vi "Grid_Scan_Stiching.vi"() -> ()   [LabVIEW 2014]
uses:
  shared/CorrelImages (SubVI)Single.vi
  <userlib>/Nanonis Prog Interface V5/Nanonis Prog Interface.lvlib
panel:
  out "Size (m) 3":cluster{"Width":sgl, "Height":sgl} {"Height" format="%.2p"; "Width" format="%.2p"}
  in  "Size (m) 2":cluster{"Width":sgl, "Height":sgl} {"Height" format="%.2p"; "Width" format="%.2p"}
  in  "Large Grid Size(m)":dbl format="%#_6p"
  in  "Tip Speed (m/s)":sgl=1e-08 format="%.2p"
  in  "Set Bias Timing (ms)":i32
  out "Grid Size 2":cluster{"Width":sgl, "Height":sgl}
  in  "Overlap (m)":dbl format="%#_6p"
  in  "Overlap (m)":cluster{"Width":sgl, "Height":sgl}
  in  "Pixels":i32 caption="Pixels/line"
  in  "Grid Coordinates":cluster{"Xc":sgl, "Yc":sgl} {"Yc" format="%.2p"; "Xc" format="%.2p"}
  out "floor(x/y)":i32
  out "yi":i32
  in  "img delay (s)":u32=1
  in  "TipLift (m)":sgl format="%#_6p"
  out "timing":i32
  out "Grid Size":cluster{"Width":sgl, "Height":sgl}
  out "Angle (deg)":sgl format="%.2f"
  out "Size (m)":cluster{"Width":sgl, "Height":sgl} {"Height" format="%.2p"; "Width" format="%.2p"}
  out "Center coordinates (m)":cluster{"Xc":sgl, "Yc":sgl} {"Yc" format="%.2p"; "Xc" format="%.2p"}
  in  "# of Grids":i32=1 min=1 max=10
  in  "ref bias":dbl=-0.0012 format="%#_6p"
  out "DC active":bool
  out "Y drift":i32
  out "X drift":i32
  in  "Current":dbl=5e-11 format="%#_6p"
  in  "Bias":dbl=0.02 format="%#_6p"
  in  "Settling time (s)":dbl=0.7 format="%#_6p"
  in  "Channel index (0-23)":u8(ring) items=["Current"=0, "Z (m)"=14]
  in  "Img Speed":sgl=4.5e-08 format="%#_6p"
  in  "Img Bias (V) DC":sgl=1.0 format="%_2p"
  in  "Img Current":sgl=1e-10 format="%#_6p"
  in  "Drift correction Pixels":i32=128
  in  "Forward Speed":sgl=1.2e-09 format="%#_6p"
  in  "Backward Speed":sgl=8e-08 format="%#_6p"
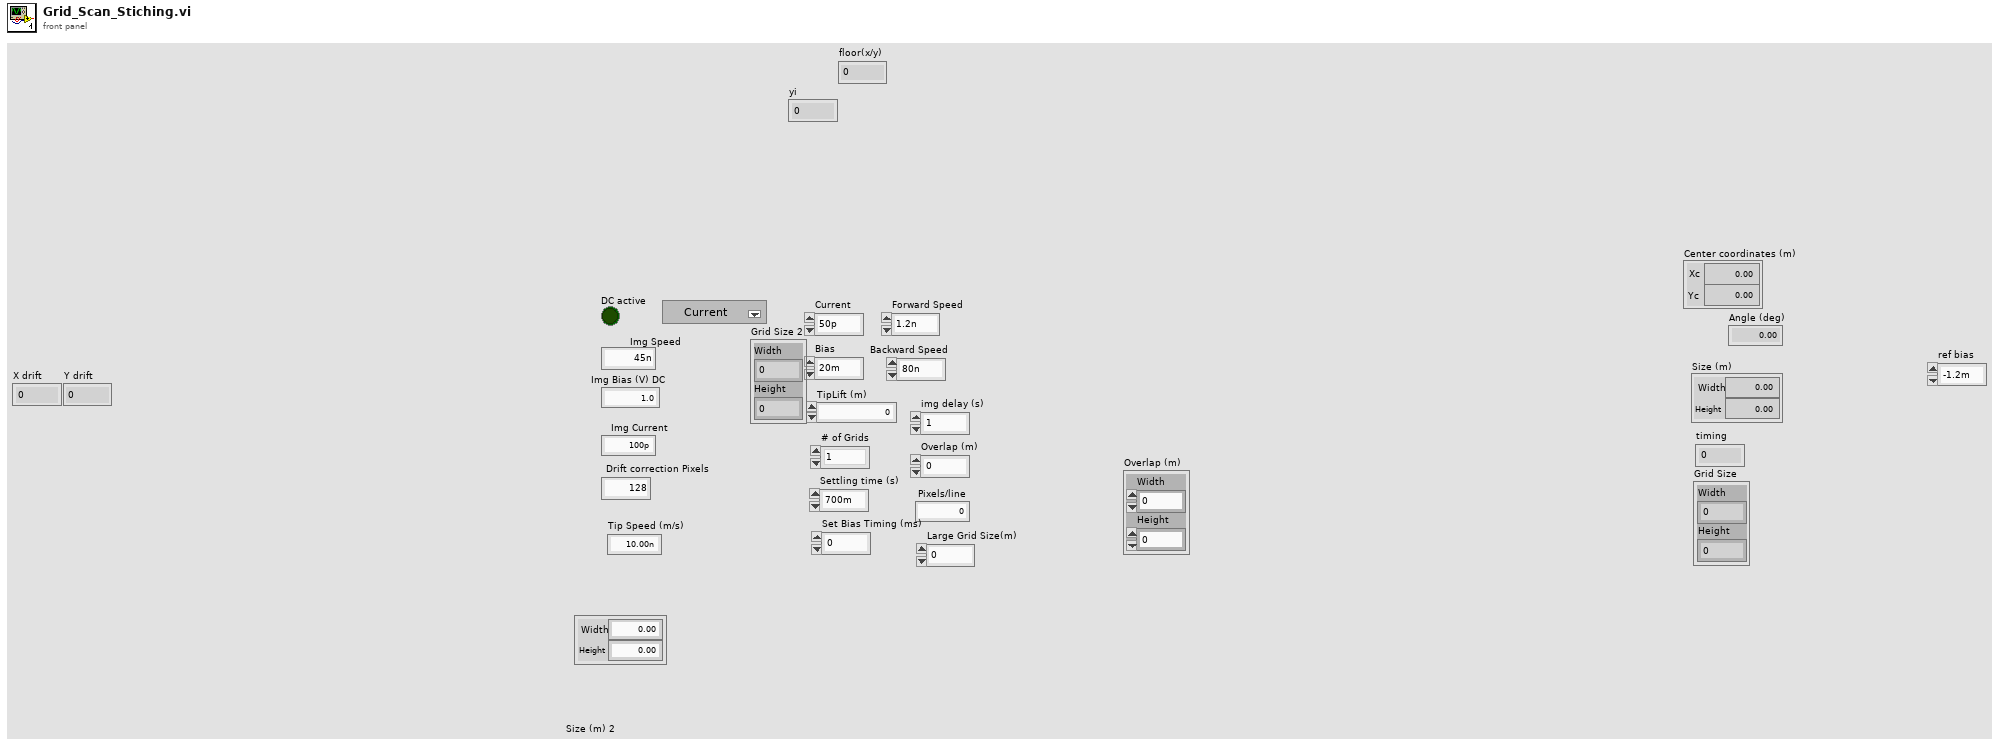
[diagram p1: front panel]
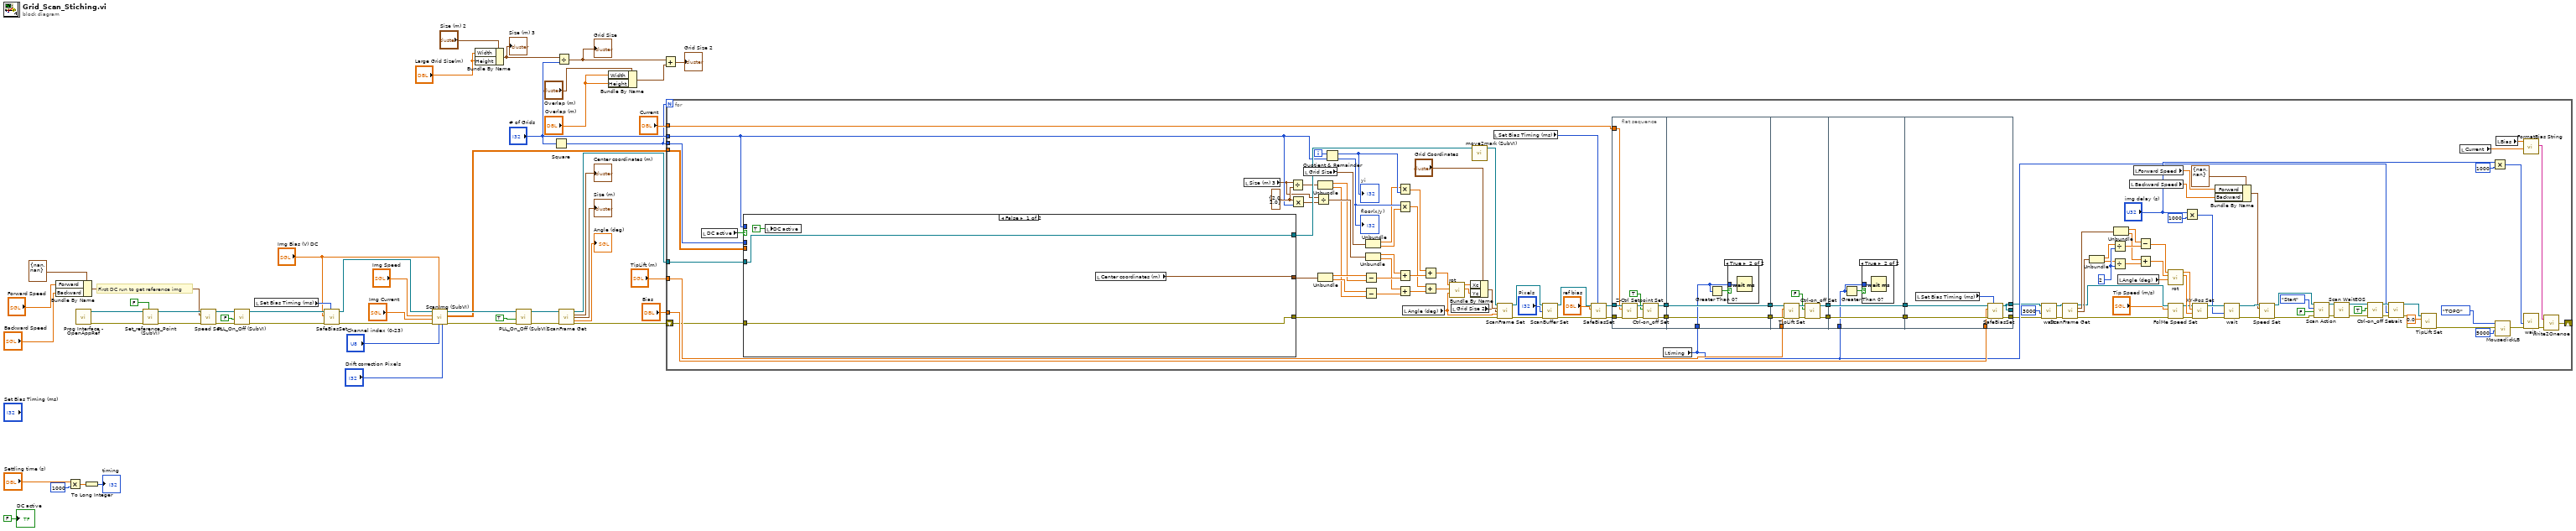
[diagram p0: block diagram]
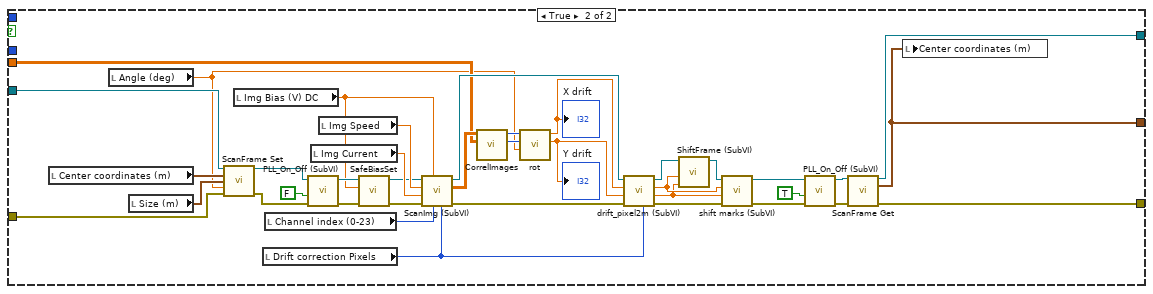
[diagram p2: hidden frame]
diagram:
  # "First DC run to get reference img"
  n1 = Bundle By Name(cluster=cluster{"Forward":sgl, "Backward":sgl} {"Forward"=nan, "Backward"=nan} ("Speed (m/s)"), "Forward"="Forward Speed", "Backward"="Backward Speed") -> (w44:cluster{"Forward":sgl, "Backward":sgl})
  n2 = Multiply(x="Settling time (s)", y=u32 1000) -> (x*y=w28:dbl)
  n3 = call <userlib>:"Prog Interface - OpenAppRef.vi"() -> ("Error out"=w50:errorcluster, "Application reference"=w51:refnum<vi>)  [unwired: 6 in]
  n4 = To Long Integer(number=w28) -> (32bit integer=→"timing":i32)
  n5 = call "Set_reference_Point (SubVI).vi"("Part of multigrid"=FALSE, "error in (no error)"=w50, "Application in"=w51) -> ("error out"=w46:errorcluster, "Application out"=w45:refnum<vi>)  [unwired: 7 in]
  n6 = call <userlib>:"Speed Set.vi"("Application ref in"=w45, "Speed (m/s)"=w44, "error in (no error)"=w46) -> ("Application ref out"=w41:refnum<vi>, "error out"=w42:errorcluster)  [unwired: 11 in]
  n7 = call "PLL_On_Off (SubVI).vi"("error in (no error)"=w42, "Output ON/OFF (F=OFF)"=FALSE, "Application in"=w41) -> ("error out"=w8:errorcluster, "Application out"=w7:refnum<vi>)  [unwired: 7 in]
  n8 = local read "Set Bias Timing (ms)"() -> (w5:i32)
  n9 = call "SafeBiasSet.vi"("Application ref in"=w7, "Bias (V)"="Img Bias (V) DC", "error in (no error)"=w8, "milliseconds to wait"=w5) -> ("Application ref out"=w6:refnum<vi>, "Error out"=w9:errorcluster)  [unwired: 5 in]
  n10 = call "ScanImg (SubVI).vi"("pixel"="Drift correction Pixels", "Channel index (0-23)"="Channel index (0-23)", "Bias (V)"="Img Bias (V) DC", "error in (no error)"=w9, "Current"="Img Current", "Img Speed"="Img Speed", "Application in"=w6) -> ("error out"=w37:errorcluster, "Img"=w10:dbl[][], "Application out"=w38:refnum<vi>)  [unwired: 2 in]
  n11 = Bundle By Name(cluster="Size (m) 2", "Width"="Large Grid Size(m)", "Height"="Large Grid Size(m)") -> (w1:cluster{"Width":sgl, "Height":sgl})
  "Size (m) 3" <- w1
  n12 = call "PLL_On_Off (SubVI).vi"("error in (no error)"=w37, "Output ON/OFF (F=OFF)"=TRUE, "Application in"=w38) -> ("error out"=w32:errorcluster, "Application out"=w33:refnum<vi>)  [unwired: 7 in]
  n13 = Square(x="# of Grids") -> (x^2=w20:i32)
  n14 = Divide(x=w1, y="# of Grids") -> (x/y=w11:cluster{"Width":sgl, "Height":sgl})
  "Grid Size" <- w11
  n15 = call <userlib>:"ScanFrame Get.vi"("Application ref in"=w33, "error in (no error)"=w32) -> ("Application ref out"=w22:refnum<vi>, "Center coordinates (m)"=→"Center coordinates (m)":cluster{"Xc":sgl, "Yc":sgl}, "Size (m)"=→"Size (m)":cluster{"Width":sgl, "Height":sgl}, "Angle (deg)"=→"Angle (deg)":sgl, "error out"=w16:errorcluster)  [unwired: 9 in]
  n16 = Bundle By Name(cluster="Overlap (m)", "Width"="Overlap (m)", "Height"="Overlap (m)") -> (w14:cluster{"Width":sgl, "Height":sgl})
  n17 = Add(x=w11, y=w14) -> (x+y=→"Grid Size 2":cluster{"Width":sgl, "Height":sgl})
  n18 = for {
    N: w20 -> [_]
    tunnel: "TipLift (m)" -> [w162]
    tunnel: "Bias" -> [w161]
    shift-right: [w70] -> _
    shift-left: w16 -> [w117]
    tunnel: "Current" -> [w119]
    tunnel: w22 -> [w115]
    tunnel: "# of Grids" -> [w110]
    tunnel: w20 -> [w114]
    tunnel: w10 -> [w52]
    i -> [w112]
    w111 = cluster{"Width":sgl, "Height":sgl} {"Width"=2.0, "Height"=2.0} ("y")
    w149 = 2
    n19 = local read "DC active"() -> (w74:bool)
    n20 = case shown="False" w74 {
      tunnel: [w176 w186] -> w118
      tunnel: w117 -> [w176 w192]
      tunnel: [w175 w193] -> w116
      tunnel: w115 -> [w175 w191]
      tunnel: w110 -> [_ _]
      tunnel: w114 -> [_ _]
      tunnel: [w174 w178] -> w97
      tunnel: w52 -> [_ w185]
      frame False {
        n21 = local write "DC active"(TRUE ("DC active")) -> ()
        n22 = local read "Center coordinates (m)"() -> (w174:cluster{"Xc":sgl, "Yc":sgl})
      }
      frame True {
        n23 = local read "Center coordinates (m)"() -> (w188:cluster{"Xc":sgl, "Yc":sgl})
        n24 = local read "Angle (deg)"() -> (w179:sgl)
        n25 = local read "Size (m)"() -> (w187:cluster{"Width":sgl, "Height":sgl})
        n26 = call <userlib>:"ScanFrame Set.vi"("Application ref in"=w191, "Center coordinates (m)"=w188, "Size (m)"=w187, "Angle (deg)"=w179, "error in (no error)"=w192) -> ("Application ref out"=w190:refnum<vi>, "error out"=w189:errorcluster)  [unwired: 9 in]
        n27 = local read "Img Bias (V) DC"() -> (w180:sgl)
        n28 = local read "Drift correction Pixels"() -> (w210:i32)
        n29 = local read "Channel index (0-23)"() -> (w206:u8)
        n30 = call "PLL_On_Off (SubVI).vi"("error in (no error)"=w189, "Output ON/OFF (F=OFF)"=FALSE, "Application in"=w190) -> ("error out"=w182:errorcluster, "Application out"=w184:refnum<vi>)  [unwired: 7 in]
        n31 = local read "Img Current"() -> (w205:sgl)
        n32 = local read "Img Speed"() -> (w204:sgl)
        n33 = call "SafeBiasSet.vi"("Application ref in"=w184, "Bias (V)"=w180, "error in (no error)"=w182) -> ("Application ref out"=w183:refnum<vi>, "Error out"=w181:errorcluster)  [unwired: 6 in]
        n34 = call "ScanImg (SubVI).vi"("pixel"=w210, "Channel index (0-23)"=w206, "Bias (V)"=w180, "error in (no error)"=w181, "Current"=w205, "Img Speed"=w204, "Application in"=w183) -> ("error out"=w215:errorcluster, "Img"=w203:dbl[][], "Application out"=w208:refnum<vi>)  [unwired: 2 in]
        n35 = call-poly "CorrelImages.vi"("Ref Array"=w185, "New Image"=w203) -> ("Y drift"=w213:i32, "X drift"=w211:i32)  [unwired: 6 in, 2 out]
        n36 = call "rot.vi"("angle"=w179, "y"=w213, "x"=w211) -> ("y'"=w214:sgl, "x'"=w212:sgl)  [unwired: 7 in]
        "X drift" <- w212
        "Y drift" <- w214
        n37 = call "drift_pixel2m (SubVI).vi"("Application in"=w208, "X drift"=w212, "Y drift"=w214, "error in"=w215, "Drift correction Pixels"=w210) -> ("Application out"=w207:refnum<vi>, "x drift"=w201:sgl, "y drift"=w200:sgl, "error out"=w199:errorcluster)  [unwired: 1 in]
        n38 = call "ShiftFrame (SubVI).vi"("Y shift"=w200, "X shift"=w201, "Application in"=w207) -> ("Application out"=w202:refnum<vi>)  [unwired: 8 in]
        n39 = call "shift marks (SubVI).vi"("error in (no error)"=w199, "y"=w200, "x"=w201, "Application in"=w202) -> ("error out"=w197:errorcluster, "Application out"=w198:refnum<vi>)  [unwired: 6 in]
        n40 = call "PLL_On_Off (SubVI).vi"("error in (no error)"=w197, "Output ON/OFF (F=OFF)"=TRUE, "Application in"=w198) -> ("error out"=w194:errorcluster, "Application out"=w195:refnum<vi>)  [unwired: 7 in]
        n41 = call <userlib>:"ScanFrame Get.vi"("Application ref in"=w195, "error in (no error)"=w194) -> ("Application ref out"=w193:refnum<vi>, "Center coordinates (m)"=w178:cluster{"Xc":sgl, "Yc":sgl}, "error out"=w186:errorcluster)  [unwired: 9 in, 2 out]
        n42 = local write "Center coordinates (m)"(w178) -> ()
      }
    }
    n43 = local read "Size (m) 3"() -> (w108:cluster{"Width":sgl, "Height":sgl})
    n44 = Divide(x=w108, y=w111) -> (x/y=w113:cluster{"Width":sgl, "Height":sgl})
    n45 = Multiply(x=w111, y=w110) -> (x*y=w109:cluster{"Width":sgl, "Height":sgl})
    n46 = local read "Grid Size"() -> (w83:cluster{"Width":sgl, "Height":sgl})
    n47 = Divide(x=w108, y=w109) -> (x/y=w107:cluster{"Width":sgl, "Height":sgl})
    n48 = Unbundle(w113) -> ("Width"=w103:sgl, "Height"=w101:sgl)
    n49 = Unbundle(w97) -> ("Xc"=w104:sgl, "Yc"=w102:sgl)
    n50 = Quotient & Remainder(x=w112, y=w110) -> (x-y*floor(x/y)=w105:i32, floor(x/y)=w106:i32)
    "yi" <- w105
    "floor(x/y)" <- w106
    n51 = Subtract(x=w104, y=w103) -> (x-y=w100:sgl)
    n52 = Subtract(x=w102, y=w101) -> (x-y=w99:sgl)
    n53 = Unbundle(w83) -> ("Width"=w82:sgl, "Height"=w81:sgl)
    n54 = Unbundle(w107) -> ("Width"=w85:sgl, "Height"=w84:sgl)
    n55 = Multiply(x=w82, y=w105) -> (x*y=w78:sgl)
    n56 = Multiply(x=w106, y=w81) -> (x*y=w75:sgl)
    n57 = Add(x=w85, y=w100) -> (x+y=w79:sgl)
    n58 = Add(x=w84, y=w99) -> (x+y=w76:sgl)
    n59 = local read "Angle (deg)"() -> (w94:sgl)
    n60 = Add(x=w78, y=w79) -> (x+y=w80:sgl)
    n61 = Add(x=w75, y=w76) -> (x+y=w77:sgl)
    n62 = call "rot.vi"("angle"=w94, "y"=w77, "x"=w80) -> ("y'"=w95:sgl, "x'"=w96:sgl)  [unwired: 7 in]
    n63 = local read "Grid Size 2"() -> (w127:cluster{"Width":sgl, "Height":sgl})
    n64 = Bundle By Name(cluster="Grid Coordinates", "Xc"=w96, "Yc"=w95) -> (w128:cluster{"Xc":sgl, "Yc":sgl})
    n65 = call "move2mark (SubVI).vi"("Application in"=w116) -> ("Application out"=w129:refnum<vi>)  [unwired: 10 in]
    n66 = local read "Set Bias Timing (ms)"() -> (w58:i32)
    n67 = call <userlib>:"ScanFrame Set.vi"("Application ref in"=w129, "Center coordinates (m)"=w128, "Size (m)"=w127, "Angle (deg)"=w94, "error in (no error)"=w118) -> ("Application ref out"=w63:refnum<vi>, "error out"=w60:errorcluster)  [unwired: 9 in]
    n68 = call <userlib>:"ScanBuffer Set.vi"("Application ref in"=w63, "Pixels"="Pixels", "error in (no error)"=w60) -> ("Application ref out"=w62:refnum<vi>, "error out"=w61:errorcluster)  [unwired: 11 in]
    n69 = call "SafeBiasSet.vi"("Application ref in"=w62, "Bias (V)"="ref bias", "error in (no error)"=w61, "milliseconds to wait"=w58) -> ("Application ref out"=w164:refnum<vi>, "Error out"=w165:errorcluster)  [unwired: 5 in]
    n70 = flat-sequence {
      tunnel: [w222] -> w173
      tunnel: [w219] -> w172
      tunnel: w164 -> [w218]
      tunnel: w165 -> [w217]
      tunnel: w119 -> [w216]
      tunnel: w173 -> [w227]
      tunnel: [w227] -> w171
      tunnel: w132 -> [w225]
      tunnel: [w224] -> w170
      tunnel: w172 -> [w224]
      tunnel: w171 -> [w236]
      tunnel: [w234] -> w169
      tunnel: w170 -> [w233]
      tunnel: [w231] -> w168
      tunnel: w162 -> [w229]
      tunnel: w169 -> [w240]
      tunnel: [w240] -> w167
      tunnel: [w238] -> w166
      tunnel: w168 -> [w238]
      tunnel: w132 -> [w237]
      tunnel: [w243] -> _
      tunnel: w167 -> [w247]
      tunnel: w166 -> [w246]
      tunnel: [w245] -> w131
      tunnel: w161 -> [w244]
      tunnel: [w243] -> w130
      frame #0 {
        n71 = call <userlib>:"Z-Ctrl Setpoint Set.vi"("error in (no error)"=w217, "Z Controller setpoint"=w216, "Application ref in"=w218) -> ("error out"=w220:errorcluster, "Application ref out"=w223:refnum<vi>)  [unwired: 7 in]
        n72 = call <userlib>:"Ctrl-on_off Set.vi"("error in (no error)"=w220, "Z Controller ON/OFF"=TRUE, "Application ref in"=w223) -> ("error out"=w219:errorcluster, "Application ref out"=w222:refnum<vi>)  [unwired: 7 in]
      }
      frame #1 {
        n73 = Greater Than 0?(x=w225) -> (x > 0?=w226:bool)
        n74 = case shown="True" w226 {
          tunnel: w225 -> [_ w228]
          frame False {
          }
          frame True {
            n75 = Wait (ms)(milliseconds to wait=w228) -> ()  [unwired: 1 out]
          }
        }
      }
      frame #2 {
        n76 = call <userlib>:"TipLift Set.vi"("error in (no error)"=w233, "TipLift (m)"=w229, "Application ref in"=w236) -> ("error out"=w232:errorcluster, "Application ref out"=w235:refnum<vi>)  [unwired: 7 in]
        n77 = call <userlib>:"Ctrl-on_off Set.vi"("error in (no error)"=w232, "Z Controller ON/OFF"=FALSE, "Application ref in"=w235) -> ("error out"=w231:errorcluster, "Application ref out"=w234:refnum<vi>)  [unwired: 7 in]
      }
      frame #3 {
        n78 = Greater Than 0?(x=w237) -> (x > 0?=w239:bool)
        n79 = case shown="True" w239 {
          tunnel: w237 -> [_ w241]
          frame False {
          }
          frame True {
            n80 = Wait (ms)(milliseconds to wait=w241) -> ()  [unwired: 1 out]
          }
        }
      }
      frame #4 {
        n81 = local read "Set Bias Timing (ms)"() -> (w242:i32)
        n82 = call "SafeBiasSet.vi"("Application ref in"=w247, "Bias (V)"=w244, "error in (no error)"=w246, "milliseconds to wait"=w242) -> ("Application ref out"=w243:refnum<vi>, "Error out"=w245:errorcluster)  [unwired: 5 in]
      }
    }
    n83 = local read "timing"() -> (w132:i32)
    n84 = call "wait.vi"("error in"=w131, "milliseconds to wait"=u32 3000 ("y"), "application reference in"=w130) -> ("error out"=w141:errorcluster, "application reference out"=w140:refnum<vi>)  [unwired: 7 in]
    n85 = call <userlib>:"ScanFrame Get.vi"("Application ref in"=w140, "error in (no error)"=w141) -> ("Application ref out"=w57:refnum<vi>, "Center coordinates (m)"=w144:cluster{"Xc":sgl, "Yc":sgl}, "Size (m)"=w145:cluster{"Width":sgl, "Height":sgl}, "error out"=w56:errorcluster)  [unwired: 9 in, 1 out]
    n86 = Unbundle(w145) -> ("Width"=w147:sgl, "Height"=w148:sgl)
    n87 = Divide(x=w147, y=w149) -> (x/y=w151:sgl)
    n88 = Divide(x=w148, y=w149) -> (x/y=w150:sgl)
    n89 = Unbundle(w144) -> ("Xc"=w152:sgl, "Yc"=w146:sgl)
    n90 = local read "Angle (deg)"() -> (w124:sgl)
    n91 = local read "Backward Speed"() -> (w87:sgl)
    n92 = local read "Forward Speed"() -> (w86:sgl)
    n93 = Subtract(x=w152, y=w151) -> (x-y=w126:sgl)
    n94 = Add(x=w146, y=w150) -> (x+y=w125:sgl)
    n95 = call "rot.vi"("angle"=w124, "y"=w125, "x"=w126) -> ("y'"=w122:sgl, "x'"=w123:sgl)  [unwired: 7 in]
    n96 = call <userlib>:"FolMe Speed Set.vi"("error in (no error)"=w56, "Speed (m/s)"="Tip Speed (m/s)", "Application ref in"=w57) -> ("error out"=w54:errorcluster, "Application ref out"=w55:refnum<vi>)  [unwired: 5 in]
    n97 = Multiply(x="img delay (s)", y=u32 1000) -> (x*y=w154:u32)
    n98 = call <userlib>:"XY-Pos Set.vi"("error in (no error)"=w54, "Y (m)"=w122, "X (m)"=w123, "Application ref in"=w55) -> ("error out"=w156:errorcluster, "Application ref out"=w155:refnum<vi>)  [unwired: 4 in]
    n99 = Bundle By Name(cluster=cluster{"Forward":sgl, "Backward":sgl} {"Forward"=nan, "Backward"=nan} ("Speed (m/s)"), "Forward"=w86, "Backward"=w87) -> (w88:cluster{"Forward":sgl, "Backward":sgl})
    n100 = call "wait.vi"("error in"=w156, "milliseconds to wait"=w154, "application reference in"=w155) -> ("error out"=w93:errorcluster, "application reference out"=w91:refnum<vi>)  [unwired: 7 in]
    n101 = call <userlib>:"Speed Set.vi"("Application ref in"=w91, "Speed (m/s)"=w88, "error in (no error)"=w93) -> ("Application ref out"=w90:refnum<vi>, "error out"=w92:errorcluster)  [unwired: 11 in]
    n102 = call <userlib>:"Scan Action.vi"("error in (no error)"=w92, "Direction: up/down (T=up)"=FALSE, "Scan action (Start)"=enum16{"Start", "Stop", "Pause", "Resume"}."Start", "Application ref in"=w90) -> ("error out"=w138:errorcluster, "Application ref out"=w139:refnum<vi>)  [unwired: 5 in]
    n103 = call <userlib>:"Scan WaitEOS.vi"("error in (no error)"=w138, "Application ref in"=w139) -> ("error out"=w120:errorcluster, "Application ref out"=w121:refnum<vi>)  [unwired: 5 in, 2 out]
    n104 = call <userlib>:"Ctrl-on_off Set.vi"("error in (no error)"=w120, "Z Controller ON/OFF"=TRUE, "Application ref in"=w121) -> ("error out"=w136:errorcluster, "Application ref out"=w134:refnum<vi>)  [unwired: 7 in]
    n105 = call "wait.vi"("error in"=w136, "milliseconds to wait"=w132, "application reference in"=w134) -> ("error out"=w135:errorcluster, "application reference out"=w133:refnum<vi>)  [unwired: 7 in]
    n106 = call <userlib>:"TipLift Set.vi"("error in (no error)"=w135, "TipLift (m)"=sgl 0.0, "Application ref in"=w133) -> ("error out"=w65:errorcluster)  [unwired: 7 in, 1 out]
    n107 = local read "Current"() -> (w68:dbl)
    n108 = Multiply(x="img delay (s)", y=u32 1000) -> (x*y=w157:u32)
    n109 = call "MouseclickLB.vi"("nMilliseconds"=5000, "error in (no error)"=w65, "Click"=enum16{"Header", "TOPO", "STS", "GRID"}."TOPO") -> ("error out"=w64:errorcluster)  [unwired: 8 in]
    n110 = local read "Bias"() -> (w69:dbl)
    n111 = call "FormatBias String.vi"("current"=w68, "bias"=w69) -> ("resulting string"=w72:string)  [unwired: 9 in]
    n112 = call "wait.vi"("error in"=w64, "milliseconds to wait"=w157) -> ("error out"=w71:errorcluster)  [unwired: 8 in, 1 out]
    n113 = call "Write2Onenoe.vi"("error in (no error)"=w71, "strSendText"=w72) -> ("error out"=w70:errorcluster)
  }
  "DC active" <- FALSE ("DC active")
